vi "Color Sensor Code.vi"() -> ()   [LabVIEW 2019]
uses:
  <vilib>/Rock Robotics/SystemInterfaces/i2clib/i2c_bus.ctl
panel:
  out "Output To Motor":dbl
  out "Color Match?":bool
  out "Matched Color Name":string
  out "Match Confidence":dbl
  out "Measured Color":cluster{"R":dbl, "G":dbl, "B":dbl}
  out "error out":errorcluster
  out "Proximity":u16(graph)
  out "Color":u32(colorbox)
  in  "Blue Calibration":cluster{"R":dbl, "G":dbl, "B":dbl}={"R"=0.143, "G"=0.427, "B"=0.429}
  in  "Green Calibration":cluster{"R":dbl, "G":dbl, "B":dbl}={"R"=0.197, "G"=0.561, "B"=0.24}
  in  "Red Calibration":cluster{"R":dbl, "G":dbl, "B":dbl}={"R"=0.561, "G"=0.323, "B"=0.114}
  in  "Yellow Calibration":cluster{"R":dbl, "G":dbl, "B":dbl}={"R"=0.361, "G"=0.524, "B"=0.113}
  in  "I2C Bus":T1
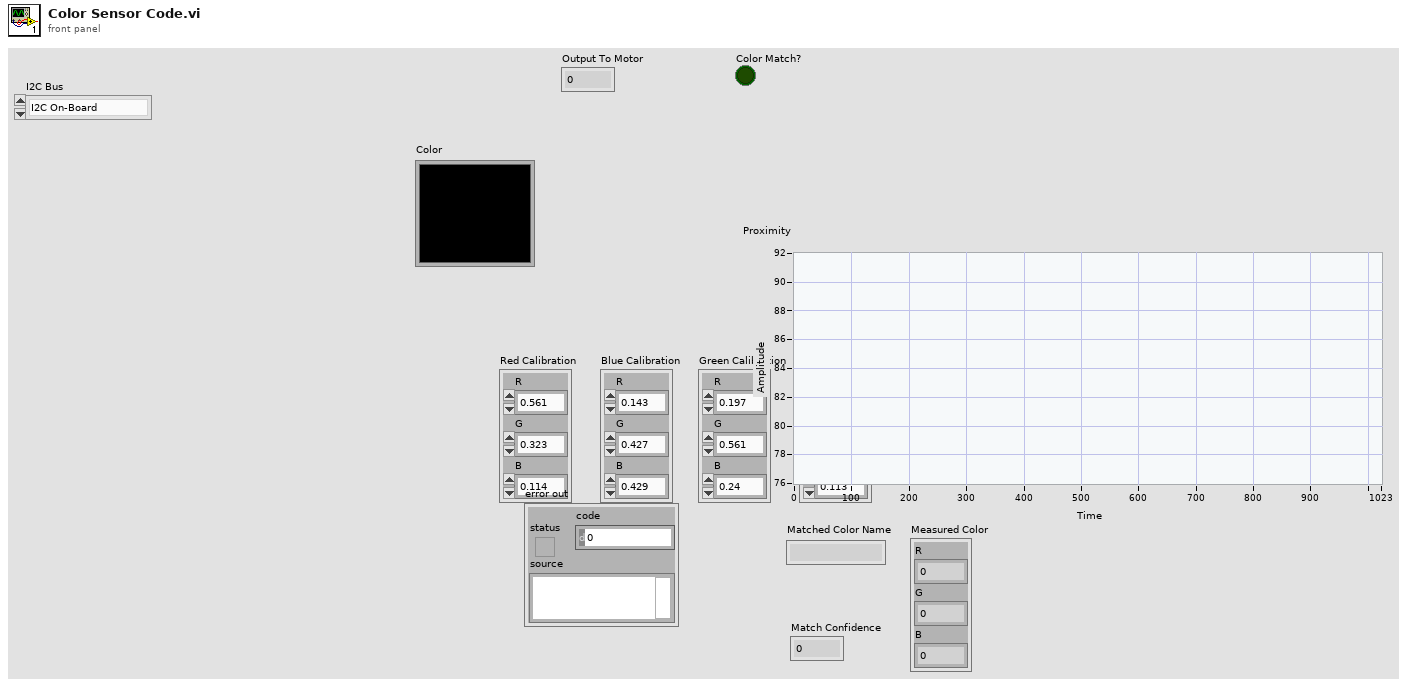
[diagram p1: front panel]
types:
  T1 = typedef "i2c_bus.ctl" = enum16{"I2C On-Board", "I2C MXP", "Invalid"}
  T2 = typedef "Color Sensor V3 DevRef.ctl" = cluster{"I2CDevRef":T3}
  T3 = typedef "WPI_I2CDevRef.ctl" = cluster{"DevStatus":errorcluster, "Device Address":u8, "Handle":i32, "I2C Bus":T1}
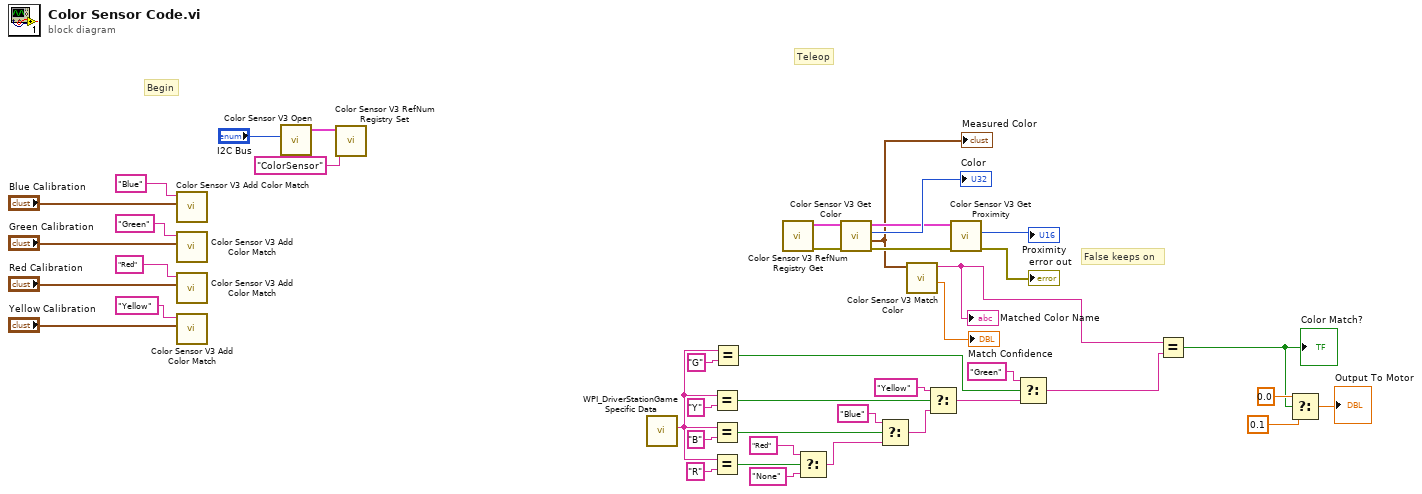
[diagram p0: block diagram]
diagram:
  # "Begin"
  # "Teleop"
  # "False keeps on"
  n1 = call <vilib>:"Color Sensor V3 Add Color Match.vi"("Color"="Blue Calibration", "Name"="Blue") -> ()  [unwired: 10 in]
  n2 = call <vilib>:"Color Sensor V3 Add Color Match.vi"("Color"="Green Calibration", "Name"="Green") -> ()  [unwired: 10 in]
  n3 = call <vilib>:"Color Sensor V3 Add Color Match.vi"("Color"="Red Calibration", "Name"="Red") -> ()  [unwired: 10 in]
  n4 = call <vilib>:"Color Sensor V3 Add Color Match.vi"("Color"="Yellow Calibration", "Name"="Yellow") -> ()  [unwired: 10 in]
  n5 = call <vilib>:"Color Sensor V3 Open.vi"("I2C Bus"="I2C Bus") -> ("ColorSensorDevRef"=w6:T2)  [unwired: 9 in, 1 out]
  n6 = call <vilib>:"Color Sensor V3 RefNum Registry Set.vi"("refnum name"="ColorSensor", "ColorSensorDevRef"=w6) -> ()  [unwired: 8 in, 2 out]
  n7 = call <vilib>:"WPI_DriverStationGame Specific Data.vi"() -> ("Game Specific Data"=w26:string)  [unwired: 11 in]
  n8 = Equal?(x=w26, y="Y") -> (x = y?=w14:bool)
  n9 = Equal?(x=w26, y="B") -> (x = y?=w18:bool)
  n10 = Equal?(x=w26, y="R") -> (x = y?=w21:bool)
  n11 = Equal?(x=w26, y="G") -> (x = y?=w11:bool)
  n12 = call <vilib>:"Color Sensor V3 RefNum Registry Get.vi"() -> ("error out"=w8:errorcluster, "ColorSensorDevRef"=w7:T2)  [unwired: 10 in]
  n13 = Select(t="Red" ("Color"), s=w21, f="None") -> (s? t:f=w17:string)
  n14 = call <vilib>:"Color Sensor V3 Get Color.vi"("error in (no error)"=w8, "ColorSensorDevRef"=w7) -> ("error out"=w33:errorcluster, "Normalized Color"=w29:cluster{"R":dbl, "G":dbl, "B":dbl}, "Color"=→"Color":u32, "ColorSensorDevRef out"=w32:T2)  [unwired: 6 in]
  "Measured Color" <- w29
  n15 = Select(t="Blue", s=w18, f=w17) -> (s? t:f=w15:string)
  n16 = call <vilib>:"Color Sensor V3 Match Color.vi"("Measured Color"=w29) -> ("Confidence"=→"Match Confidence":dbl, "Matched Color Name"=w27:string)  [unwired: 8 in, 1 out]
  "Matched Color Name" <- w27
  n17 = Select(t="Yellow", s=w14, f=w15) -> (s? t:f=w12:string)
  n18 = call <vilib>:"Color Sensor V3 Get Proximity.vi"("error in (no error)"=w33, "ColorSensorDevRef"=w32) -> ("error out"=→"error out":errorcluster, "Proximity"=→"Proximity":u16)  [unwired: 7 in, 1 out]
  n19 = Select(t="Green", s=w11, f=w12) -> (s? t:f=w9:string)
  n20 = Equal?(x=w27, y=w9) -> (x = y?=w2:bool)
  "Color Match?" <- w2
  n21 = Select(t=0.0, s=w2, f=0.1 ("Output")) -> (s? t:f=→"Output To Motor":dbl)
